vi "S2C_VLFT10_Proc_TriverseSliderSelect.vi"(8 "Error In":errorcluster, 11 "SliderSelect":string) -> (0 "Error Out":errorcluster, 3 "Result":string)   [LabVIEW 2015]
uses:
  PCIe7841/VIs/Typedefs/S2C_PCIe7841_Type_Triverse.ctl
  PCIe7841/VIs/PolyDriver/S2C_PCIe7841_Poly_TriverseWrite.vi
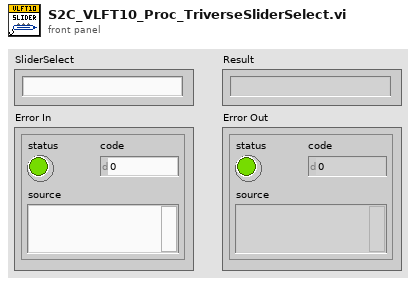
[diagram p1: front panel]
types:
  T1 = typedef "S2C_PCIe7841_Type_Triverse.ctl" = string
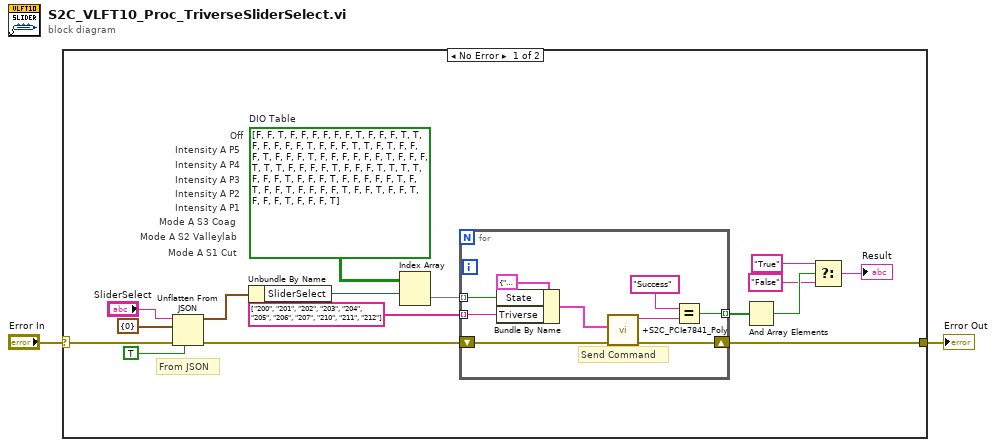
[diagram p0: block diagram]
diagram:
  n1 = case shown="No Error" "Error In" {
    selector: "Error In" -> [w6 w28]
    tunnel: [w15 w28] -> w2
    frame No Error {
      w17 = bool[][] [[FALSE, FALSE, TRUE, FALSE, FALSE, FALSE, FALSE, FALSE, FALSE, TRUE, FALSE], [FALSE, FALSE, TRUE, TRUE, FALSE, FALSE, FALSE, FALSE, FALSE, TRUE, FALSE], [FALSE, FALSE, TRUE, TRUE, FALSE, TRUE, FALSE, FALSE, FALSE, TRUE, FALSE], [FALSE, FALSE, TRUE, FALSE, FALSE, FALSE, FALSE, FALSE, FALSE, TRUE, FALSE], [FALSE, FALSE, TRUE, TRUE, TRUE, FALSE, FALSE, FALSE, FALSE, TRUE, FALSE], [FALSE, FALSE, TRUE, TRUE, TRUE, TRUE, FALSE, FALSE, FALSE, TRUE, FALSE], [FALSE, FALSE, TRUE, FALSE, FALSE, FALSE, FALSE, FALSE, TRUE, FALSE, TRUE], [FALSE, FALSE, TRUE, FALSE, FALSE, FALSE, FALSE, TRUE, FALSE, FALSE, TRUE], [FALSE, FALSE, TRUE, FALSE, FALSE, FALSE, TRUE, FALSE, FALSE, FALSE, TRUE]]  # DIO Table
      # "Mode A S1 Cut"
      # "Mode A S2 Valleylab"
      # "Mode A S3 Coag"
      # "Intensity A P1"
      # "Intensity A P2"
      # "Intensity A P3"
      # "Intensity A P4"
      # "Intensity A P5"
      # "Off"
      # "From JSON"
      n2 = Unflatten From JSON(JSON string="SliderSelect", type and defaults=cluster{"SliderSelect":u16} {"SliderSelect"=0}, default null elements? (F)=TRUE, error in (no error)=w6) -> (value=w7:cluster{"SliderSelect":u16}, error out=w4:errorcluster)  [unwired: 3 in]
      n3 = Unbundle By Name(w7) -> ("SliderSelect"=w5:u16)
      n4 = Index Array(array=w17, index (row)=w5) -> (element=w16:bool[])  [unwired: 1 in]
      n5 = for {
        tunnel: T1[] ["200", "201", "202", "203", "204", "205", "206", "207", "210", "211", "212"] -> [w25] mode=indexing
        tunnel: w16 -> [w24] mode=indexing
        shift-right: [w23] -> w15
        shift-left: w4 -> [w27]
        tunnel: [w20] -> w13 mode=indexing
        # "Send Command"
        n6 = Bundle By Name(cluster=cluster{"Triverse":T1, "State":bool} {"Triverse"="201", "State"=FALSE} ("Triverse"), "State"=w24, "Triverse"=w25) -> (w19:cluster{"Triverse":T1, "State":bool})
        n7 = call-poly "+S2C_PCIe7841_Poly.vi"("Error In"=w27, "Triverse"=w19) -> ("Error Out"=w23:errorcluster, "Response"=w22:string)  [unwired: 8 in]
        n8 = Equal?(x="Success", y=w22) -> (x = y?=w20:bool)
      }
      n9 = And Array Elements(Boolean array=w13) -> (logical AND=w12:bool)
      n10 = Select(t="True", s=w12, f="False") -> (s? t:f=→"Result":string)
    }
    frame Error {
    }
  }
  "Error Out" <- w2
